vi "SentinelController v35 good v11.vi"() -> ()   [LabVIEW 2011] (continued)
                  n306 = local write "H1 Lock"(FALSE ("H1 Lock")) -> ()
                  n307 = local write "H2 warning 2"(FALSE ("H1 warning")) -> ()
                  n308 = local write "H2 warning"(FALSE ("H1 warning")) -> ()
                  n309 = local write "H1 warning 2"(FALSE ("H1 warning")) -> ()
                  n310 = local write "H1 warning"(FALSE ("H1 warning")) -> ()
                  n311 = local write "H2 nominal 2"(TRUE ("H1 nominal")) -> ()
                  n312 = local write "H2 alarm 2"(FALSE ("H1 warning")) -> ()
                  n313 = local write "H2 alarm"(FALSE ("H1 warning")) -> ()
                  n314 = local write "H1 nominal 2"(TRUE ("H1 nominal")) -> ()
                  n315 = local write "H1 alarm 2"(FALSE ("H1 warning")) -> ()
                  n316 = local write "system statuts hid"(T9."H1NH2N" ("system statuts")) -> ()
                  n317 = local write "H1 Good Units"(w3224) -> ()
                  n318 = local write "H2 Device Count"(w3224) -> ()
                  n319 = local write "H2 Good Units"(w3224) -> ()
                  n320 = local write "H1 Device Count"(w3224) -> ()
                  n321 = property on="System UPH" class="Knob (strict)"("Scale.Minimum"=w3221) -> ()  [unwired: 2 in, 2 out]
                  n322 = property on="H1 UPH" class="Knob (strict)"("Scale.Minimum"=w3221) -> ()  [unwired: 2 in, 2 out]
                  n323 = property on="H2 UPH" class="Knob (strict)"("Scale.Minimum"=w3221) -> ()  [unwired: 2 in, 2 out]
                  n324 = property on="SysUtilMon" class="WFChart (strict)"("History Data"=cluster{dbl, dbl}[] []) -> ()  [unwired: 2 in, 2 out]
                  n325 = local write "H1 alarm"(w3239) -> ()
                  n326 = local write "H2 alarm"(w3239) -> ()
                  n327 = property on="YieldMon" class="WFChart (strict)"("History Data"=cluster{dbl, dbl, dbl, dbl}[] []) -> ()  [unwired: 2 in, 2 out]
                  n328 = local write "YieldMon"(w3216) -> ()
                  n329 = local write "SysUtilMon"(w3215) -> ()
                  n330 = local write "Sys utilization"(0.0) -> ()
                  n331 = local write "H2 alarm 2"(w3239) -> ()
                  n332 = local write "H1 alarm 2"(w3239) -> ()
                  n333 = local write "H2 nominal"(TRUE ("H1 nominal")) -> ()
                  n334 = local write "H1 nominal"(TRUE ("H1 nominal")) -> ()
                  n335 = local read "Lot number"() -> (w3213:string)
                  n336 = local write "Number of text alerts"(0.0 ("Number of Emails Alerts Sent")) -> ()
                  n337 = local write "Number of email alerts"(u32 0 ("Number of Emails Alerts Sent")) -> ()
                  n338 = local write "Tester loop counter hid"(u32 0 ("Tester loop counter")) -> ()
                  n339 = local write "H1 loop counter hid"(u32 0 ("H1 loop counter hid")) -> ()
                  n340 = local write "H2 loop counter hid"(u32 0 ("H2 loop counter hid")) -> ()
                  n341 = local write "H1 Ready with sites"(FALSE ("H1 Ready with sites")) -> ()
                  n342 = local write "H2 Ready with sites"(FALSE ("H1 Ready with sites")) -> ()
                  n343 = local write "GPIB Bus 0 traffic"(w3218) -> ()
                  n344 = local write "Notifications Lot Display"(w3213) -> ()
                  n345 = local write "GPIB bus 1 traffic"(w3218) -> ()
                  n346 = local write "GPIB bus 2 traffic"(w3218) -> ()
                }
              }
              n347 = case shown="True" w3122 {
                frame False {
                }
                frame True {
                  w3198 = FALSE
                  n348 = local read "H1 online"() -> (w3200:bool)
                  n349 = local read "H2 online"() -> (w3199:bool)
                  n350 = Equal?(x=w3200, y=w3198) -> (x = y?=w3202:bool)
                  n351 = Equal?(x=w3198, y=w3199) -> (x = y?=w3201:bool)
                  n352 = Or(x=w3202, y=w3201) -> (x .or. y?=w3197:bool)
                  n353 = case shown="True" w3197 {
                    frame False {
                    }
                    frame True {
                      n354 = local write "Optimize handler speed"(FALSE ("Optimize Handler Speed")) -> ()
                    }
                  }
                }
              }
              n355 = local read "Alert volume"() -> (w3133:u32)
              n356 = Equal To 0?(x=w3133) -> (x = 0?=w3135:bool)
              n357 = case shown="True" w3135 {
                frame False {
                }
                frame True {
                  n358 = local write "Audio On / Off"(FALSE ("Audio On/Off")) -> ()
                }
              }
            }
            n359 = case shown="True" FALSE {
              frame False {
              }
              frame True {
                n360 = while {
                  i -> [w952]
                  stop <- w965 stop-if-true
                  # "Play Audio Aert Loop"
                  n361 = local read "Ignore alarms until AFTER this many cycles"() -> (w957:i32)
                  n362 = local read "H1 Device Count"() -> (w962:u32)
                  n363 = local read "H2 Device Count"() -> (w961:u32)
                  n364 = local read "Program Parallelism"() -> (w959:u32)
                  n365 = local read "Run"() -> (w954:bool)
                  n366 = local read "POWER"() -> (w955:bool)
                  n367 = Add(x=w962, y=w961) -> (x+y=w960:u32)
                  n368 = Wait (ms)(milliseconds to wait=u32 100) -> ()  [unwired: 1 out]
                  n369 = Divide(x=w960, y=w959) -> (x/y=w958:dbl)
                  n370 = Greater?(x=w952, y=50) -> (0:w950:bool)
                  n371 = Greater?(x=w958, y=w957) -> (0:w956:bool)
                  n372 = Compound Arithmetic op=AND(w956, w955, w954, w950) -> (w953:bool)
                  n373 = case shown="True" w953 {
                    frame False {
                    }
                    frame True {
                      n374 = local read "system statuts hid"() -> (w969:T9)
                      n375 = case shown="\"H1AH2A\"" w969 {
                        frame "H1NH2N", Default {
                          n376 = Wait (ms)(milliseconds to wait=u32 50) -> ()  [unwired: 1 out]
                        }
                        frame "H1NH2W" {
                          n377 = flat-sequence {
                            frame #0 {
                              n378 = local read "Audio On / Off"() -> (w972:bool)
                              n379 = local read "H2 online"() -> (w971:bool)
                              n380 = And(x=w971, y=w972) -> (x .and. y?=w973:bool)
                              n381 = case shown="True" w973 {
                                frame False {
                                }
                                frame True {
                                n382 = local read "Run"() -> (w976:bool)
                                n383 = case shown="True" w976 {
                                tunnel: [0.001 w978] -> w975
                                frame False {
                                }
                                frame True {
                                n384 = local read "Alert volume"() -> (w978:u32)
                                }
                                }
                                n385 = call "PlayAlarm.vi"("wavefilename"="audio\\4_synth_warning.wav", "alertvolume"=w975) -> ()  [unwired: 10 in]
                                }
                              }
                            }
                            frame #1 {
                              n386 = local read "Run"() -> (w979:bool)
                              n387 = case shown="True" w979 {
                                frame False {
                                }
                                frame True {
                                n388 = Wait (ms)(milliseconds to wait=u32 5000) -> ()  [unwired: 1 out]
                                }
                              }
                            }
                          }
                        }
                        frame "H1NH2A" {
                          n389 = flat-sequence {
                            frame #0 {
                              n390 = local read "Audio On / Off"() -> (w983:bool)
                              n391 = local read "H2 online"() -> (w982:bool)
                              n392 = And(x=w982, y=w983) -> (x .and. y?=w981:bool)
                              n393 = case shown="True" w981 {
                                frame False {
                                }
                                frame True {
                                n394 = local read "Run"() -> (w986:bool)
                                n395 = case shown="True" w986 {
                                tunnel: [0.001 w988] -> w985
                                frame False {
                                }
                                frame True {
                                n396 = local read "Alert volume"() -> (w988:u32)
                                }
                                }
                                n397 = call "PlayAlarm.vi"("wavefilename"="audio\\bass_synth_alarm.wav", "alertvolume"=w985) -> ()  [unwired: 10 in]
                                }
                              }
                            }
                            frame #1 {
                              n398 = local read "Run"() -> (w989:bool)
                              n399 = case shown="True" w989 {
                                frame False {
                                n400 = Wait (ms)(milliseconds to wait=u32 50) -> ()  [unwired: 1 out]
                                }
                                frame True {
                                n401 = Wait (ms)(milliseconds to wait=u32 5000) -> ()  [unwired: 1 out]
                                }
                              }
                            }
                          }
                        }
                        frame "H1WH2N" {
                          n402 = flat-sequence {
                            frame #0 {
                              n403 = local read "Audio On / Off"() -> (w994:bool)
                              n404 = local read "H1 online"() -> (w993:bool)
                              n405 = And(x=w993, y=w994) -> (x .and. y?=w992:bool)
                              n406 = case shown="True" w992 {
                                frame False {
                                }
                                frame True {
                                n407 = local read "Run"() -> (w997:bool)
                                n408 = case shown="True" w997 {
                                tunnel: [0.001 w999] -> w996
                                frame False {
                                }
                                frame True {
                                n409 = local read "Alert volume"() -> (w999:u32)
                                }
                                }
                                n410 = call "PlayAlarm.vi"("wavefilename"="audio\\4_synth_warning.wav", "alertvolume"=w996) -> ()  [unwired: 10 in]
                                }
                              }
                            }
                            frame #1 {
                              n411 = local read "Run"() -> (w1000:bool)
                              n412 = case shown="True" w1000 {
                                frame False {
                                n413 = Wait (ms)(milliseconds to wait=u32 50) -> ()  [unwired: 1 out]
                                }
                                frame True {
                                n414 = Wait (ms)(milliseconds to wait=u32 5000) -> ()  [unwired: 1 out]
                                }
                              }
                            }
                          }
                        }
                        frame "H1WH2W" {
                          n415 = flat-sequence {
                            frame #0 {
                              n416 = local read "Audio On / Off"() -> (w1006:bool)
                              n417 = local read "H1 online"() -> (w1003:bool)
                              n418 = local read "H2 online"() -> (w1005:bool)
                              n419 = Compound Arithmetic op=AND(w1003, w1005, w1006) -> (w1004:bool)
                              n420 = case shown="True" w1004 {
                                frame False {
                                }
                                frame True {
                                n421 = local read "Run"() -> (w1009:bool)
                                n422 = case shown="True" w1009 {
                                tunnel: [0.001 w1011] -> w1008
                                frame False {
                                }
                                frame True {
                                n423 = local read "Alert volume"() -> (w1011:u32)
                                }
                                }
                                n424 = call "PlayAlarm.vi"("wavefilename"="audio\\4_synth_warning.wav", "alertvolume"=w1008) -> ()  [unwired: 10 in]
                                }
                              }
                            }
                            frame #1 {
                              n425 = local read "Run"() -> (w1012:bool)
                              n426 = case shown="True" w1012 {
                                frame False {
                                n427 = Wait (ms)(milliseconds to wait=u32 50) -> ()  [unwired: 1 out]
                                }
                                frame True {
                                n428 = Wait (ms)(milliseconds to wait=u32 5000) -> ()  [unwired: 1 out]
                                }
                              }
                            }
                          }
                        }
                        frame "H1WH2A" {
                          n429 = flat-sequence {
                            frame #0 {
                              n430 = local read "Audio On / Off"() -> (w1018:bool)
                              n431 = local read "H1 online"() -> (w1016:bool)
                              n432 = local read "H2 online"() -> (w1017:bool)
                              n433 = Compound Arithmetic op=AND(w1016, w1017, w1018) -> (w1015:bool)
                              n434 = case shown="True" w1015 {
                                frame False {
                                }
                                frame True {
                                n435 = local read "Run"() -> (w1021:bool)
                                n436 = case shown="True" w1021 {
                                tunnel: [0.001 w1023] -> w1020
                                frame False {
                                }
                                frame True {
                                n437 = local read "Alert volume"() -> (w1023:u32)
                                }
                                }
                                n438 = call "PlayAlarm.vi"("wavefilename"="audio\\bass_synth_alarm.wav", "alertvolume"=w1020) -> ()  [unwired: 10 in]
                                }
                              }
                            }
                            frame #1 {
                              n439 = local read "Run"() -> (w1024:bool)
                              n440 = case shown="True" w1024 {
                                frame False {
                                n441 = Wait (ms)(milliseconds to wait=u32 50) -> ()  [unwired: 1 out]
                                }
                                frame True {
                                n442 = Wait (ms)(milliseconds to wait=u32 5000) -> ()  [unwired: 1 out]
                                }
                              }
                            }
                          }
                        }
                        frame "H1AH2N" {
                          n443 = flat-sequence {
                            frame #0 {
                              n444 = local read "Audio On / Off"() -> (w1029:bool)
                              n445 = local read "H1 online"() -> (w1027:bool)
                              n446 = And(x=w1027, y=w1029) -> (x .and. y?=w1028:bool)
                              n447 = case shown="True" w1028 {
                                frame False {
                                }
                                frame True {
                                n448 = local read "Run"() -> (w1032:bool)
                                n449 = case shown="True" w1032 {
                                tunnel: [0.001 w1034] -> w1031
                                frame False {
                                }
                                frame True {
                                n450 = local read "Alert volume"() -> (w1034:u32)
                                }
                                }
                                n451 = call "PlayAlarm.vi"("wavefilename"="audio\\bass_synth_alarm.wav", "alertvolume"=w1031) -> ()  [unwired: 10 in]
                                }
                              }
                            }
                            frame #1 {
                              n452 = local read "Run"() -> (w1035:bool)
                              n453 = case shown="True" w1035 {
                                frame False {
                                n454 = Wait (ms)(milliseconds to wait=u32 50) -> ()  [unwired: 1 out]
                                }
                                frame True {
                                n455 = Wait (ms)(milliseconds to wait=u32 5000) -> ()  [unwired: 1 out]
                                }
                              }
                            }
                          }
                        }
                        frame "H1AH2W" {
                          n456 = flat-sequence {
                            frame #0 {
                              n457 = local read "Audio On / Off"() -> (w1041:bool)
                              n458 = local read "H1 online"() -> (w1039:bool)
                              n459 = local read "H2 online"() -> (w1040:bool)
                              n460 = Compound Arithmetic op=AND(w1039, w1040, w1041) -> (w1038:bool)
                              n461 = case shown="True" w1038 {
                                frame False {
                                }
                                frame True {
                                n462 = local read "Run"() -> (w1044:bool)
                                n463 = case shown="True" w1044 {
                                tunnel: [0.001 w1046] -> w1043
                                frame False {
                                }
                                frame True {
                                n464 = local read "Alert volume"() -> (w1046:u32)
                                }
                                }
                                n465 = call "PlayAlarm.vi"("wavefilename"="audio\\bass_synth_alarm.wav", "alertvolume"=w1043) -> ()  [unwired: 10 in]
                                }
                              }
                            }
                            frame #1 {
                              n466 = local read "Run"() -> (w1047:bool)
                              n467 = case shown="True" w1047 {
                                frame False {
                                n468 = Wait (ms)(milliseconds to wait=u32 50) -> ()  [unwired: 1 out]
                                }
                                frame True {
                                n469 = Wait (ms)(milliseconds to wait=u32 5000) -> ()  [unwired: 1 out]
                                }
                              }
                            }
                          }
                        }
                        frame "H1AH2A" {
                          n470 = flat-sequence {
                            frame #0 {
                              n471 = local read "Audio On / Off"() -> (w1053:bool)
                              n472 = local read "H1 online"() -> (w1051:bool)
                              n473 = local read "H2 online"() -> (w1052:bool)
                              n474 = Compound Arithmetic op=AND(w1051, w1052, w1053) -> (w1050:bool)
                              n475 = case shown="True" w1050 {
                                frame False {
                                }
                                frame True {
                                n476 = local read "Run"() -> (w1056:bool)
                                n477 = case shown="True" w1056 {
                                tunnel: [0.001 w1058] -> w1055
                                frame False {
                                }
                                frame True {
                                n478 = local read "Alert volume"() -> (w1058:u32)
                                }
                                }
                                n479 = call "PlayAlarm.vi"("wavefilename"="audio\\bass_synth_alarm.wav", "alertvolume"=w1055) -> ()  [unwired: 10 in]
                                }
                              }
                            }
                            frame #1 {
                              n480 = local read "Run"() -> (w1059:bool)
                              n481 = case shown="True" w1059 {
                                frame False {
                                n482 = Wait (ms)(milliseconds to wait=u32 50) -> ()  [unwired: 1 out]
                                }
                                frame True {
                                n483 = Wait (ms)(milliseconds to wait=u32 5000) -> ()  [unwired: 1 out]
                                }
                              }
                            }
                          }
                        }
                      }
                    }
                  }
                  n484 = local read "Run"() -> (w963:bool)
                  n485 = local read "POWER"() -> (w966:bool)
                  n486 = Not(x=w966) -> (.not. x?=w968:bool)
                  n487 = Not(x=w963) -> (.not. x?=w967:bool)
                  n488 = Compound Arithmetic op=OR(w968, w967) -> (w965:bool)
                }
              }
            }
            n489 = while {
              shift-right: [w2528] -> _
              shift-left: T9."H1NH2N" ("system statuts") -> [w2518]
              stop <- w2517 continue-if-true
              # "system status state machine:\n- writes data log whenever there is a change (if data loggin enabled)\n- issues email and text alerts is enabled (electronic notification of alarms)"
              n490 = local read "H1 parallelism"() -> (w2524:u32)
              n491 = local read "H1 Device Count"() -> (w2525:u32)
              n492 = local read "H2 Device Count"() -> (w2523:u32)
              n493 = local read "H2 parallelism"() -> (w2522:u32)
              n494 = local read "POWER"() -> (w2517:bool)
              n495 = Divide(x=w2523, y=w2522) -> (x/y=w2519:dbl)
              n496 = Divide(x=w2525, y=w2524) -> (x/y=w2520:dbl)
              n497 = local read "Ignore alarms until AFTER this many cycles"() -> (w2527:i32)
              n498 = Add(x=w2520, y=w2519) -> (x+y=w2521:dbl)
              n499 = Greater?(x=w2521, y=w2527) -> (0:w2526:bool)
              n500 = case shown="True" w2526 {
                tunnel: [w2530 w2533] -> w2528
                tunnel: w2518 -> [w2530 w2531]
                frame False {
                }
                frame True {
                  n501 = flat-sequence {
                    tunnel: [w2534] -> w2532
                    tunnel: w2531 -> [w2534]
                    tunnel: [w2631] -> w2533
                    tunnel: w2532 -> [w2629]
                    frame #0 {
                      # "Determine current state for System Status state-machine"
                      n502 = stacked-sequence {
                        frame #0 {
                          n503 = local read "H1 nominal 2"() -> (w2538:bool)
                          n504 = local read "H2 nominal 2"() -> (w2536:bool)
                          n505 = local read "H1 nominal"() -> (w2539:bool)
                          n506 = local read "H2 nominal"() -> (w2537:bool)
                          n507 = Compound Arithmetic op=AND(w2539, w2538, w2537, w2536) -> (w2535:bool)
                          n508 = case shown="True" w2535 {
                            frame False {
                            }
                            frame True {
                              n509 = local write "system statuts hid"(T9."H1NH2N" ("system statuts")) -> ()
                            }
                          }
                        }
                        frame #1 {
                          n510 = local read "H2 warning 2"() -> (w2543:bool)
                          n511 = local read "H2 warning"() -> (w2544:bool)
                          n512 = local read "H1 nominal 2"() -> (w2545:bool)
                          n513 = local read "H1 nominal"() -> (w2546:bool)
                          n514 = Or(x=w2544, y=w2543) -> (x .or. y?=w2542:bool)
                          n515 = Compound Arithmetic op=AND(w2546, w2545, w2542) -> (w2541:bool)
                          n516 = case shown="False" w2541 {
                            frame False {
                            }
                            frame True {
                              n517 = local write "system statuts hid"(T9."H1NH2W" ("system statuts")) -> ()
                            }
                          }
                        }
                        frame #2 {
                          n518 = local read "H1 nominal 2"() -> (w2553:bool)
                          n519 = local read "H1 nominal"() -> (w2554:bool)
                          n520 = local read "H2 alarm 2"() -> (w2551:bool)
                          n521 = local read "H2 alarm"() -> (w2552:bool)
                          n522 = Or(x=w2552, y=w2551) -> (x .or. y?=w2549:bool)
                          n523 = And(x=w2554, y=w2553) -> (x .and. y?=w2550:bool)
                          n524 = And(x=w2550, y=w2549) -> (x .and. y?=w2548:bool)
                          n525 = case shown="True" w2548 {
                            frame False {
                            }
                            frame True {
                              n526 = local write "system statuts hid"(T9."H1NH2A" ("system statuts")) -> ()
                            }
                          }
                        }
                        frame #3 {
                          n527 = local read "H1 alarm 2"() -> (w2564:bool)
                          n528 = local read "H1 alarm"() -> (w2565:bool)
                          n529 = local read "H2 nominal 2"() -> (w2567:bool)
                          n530 = local read "H1 warning 2"() -> (w2560:bool)
                          n531 = local read "H1 warning"() -> (w2561:bool)
                          n532 = local read "H2 nominal"() -> (w2566:bool)
                          n533 = Not(x=w2565) -> (.not. x?=w2563:bool)
                          n534 = Not(x=w2564) -> (.not. x?=w2562:bool)
                          n535 = Or(x=w2561, y=w2560) -> (x .or. y?=w2558:bool)
                          n536 = And(x=w2563, y=w2562) -> (x .and. y?=w2557:bool)
                          n537 = And(x=w2566, y=w2567) -> (x .and. y?=w2556:bool)
                          n538 = Compound Arithmetic op=AND(w2558, w2557, w2556) -> (w2559:bool)
                          n539 = case shown="True" w2559 {
                            frame False {
                            }
                            frame True {
                              n540 = local write "system statuts hid"(T9."H1WH2N" ("system statuts")) -> ()
                            }
                          }
                        }
                        frame #4 {
                          n541 = local read "H1 alarm 2"() -> (w2579:bool)
                          n542 = local read "H2 alarm 2"() -> (w2584:bool)
                          n543 = local read "H1 alarm"() -> (w2578:bool)
                          n544 = local read "H2 alarm"() -> (w2585:bool)
                          n545 = local read "H1 warning 2"() -> (w2575:bool)
                          n546 = local read "H2 warning 2"() -> (w2576:bool)
                          n547 = local read "H1 warning"() -> (w2574:bool)
                          n548 = local read "H2 warning"() -> (w2577:bool)
                          n549 = Not(x=w2578) -> (.not. x?=w2580:bool)
                          n550 = Not(x=w2579) -> (.not. x?=w2581:bool)
                          n551 = Not(x=w2585) -> (.not. x?=w2583:bool)
                          n552 = Not(x=w2584) -> (.not. x?=w2582:bool)
                          n553 = Or(x=w2574, y=w2575) -> (x .or. y?=w2572:bool)
                          n554 = Or(x=w2577, y=w2576) -> (x .or. y?=w2570:bool)
                          n555 = And(x=w2580, y=w2581) -> (x .and. y?=w2571:bool)
                          n556 = And(x=w2583, y=w2582) -> (x .and. y?=w2569:bool)
                          n557 = Compound Arithmetic op=AND(w2572, w2571, w2570, w2569) -> (w2573:bool)
                          n558 = case shown="True" w2573 {
                            frame False {
                            }
                            frame True {
                              n559 = local write "system statuts hid"(T9."H1WH2W" ("system statuts")) -> ()
                            }
                          }
                        }
                        frame #5 {
                          n560 = local read "H1 alarm 2"() -> (w2592:bool)
                          n561 = local read "H1 alarm"() -> (w2593:bool)
                          n562 = local read "H1 warning 2"() -> (w2595:bool)
                          n563 = local read "H1 warning"() -> (w2596:bool)
                          n564 = local read "H2 alarm 2"() -> (w2597:bool)
                          n565 = local read "H2 alarm"() -> (w2598:bool)
                          n566 = Not(x=w2593) -> (.not. x?=w2591:bool)
                          n567 = Not(x=w2592) -> (.not. x?=w2590:bool)
                          n568 = Or(x=w2596, y=w2595) -> (x .or. y?=w2589:bool)
                          n569 = Or(x=w2598, y=w2597) -> (x .or. y?=w2587:bool)
                          n570 = And(x=w2591, y=w2590) -> (x .and. y?=w2588:bool)
                          n571 = Compound Arithmetic op=AND(w2589, w2588, w2587) -> (w2594:bool)
                          n572 = case shown="True" w2594 {
                            frame False {
                            }
                            frame True {
                              n573 = local write "system statuts hid"(T9."H1WH2A" ("system statuts")) -> ()
                            }
                          }
                        }
                        frame #6 {
                          n574 = local read "H2 nominal 2"() -> (w2605:bool)
                          n575 = local read "H2 nominal"() -> (w2606:bool)
                          n576 = local read "H1 alarm 2"() -> (w2603:bool)
                          n577 = local read "H1 alarm"() -> (w2604:bool)
                          n578 = Or(x=w2604, y=w2603) -> (x .or. y?=w2601:bool)
                          n579 = And(x=w2606, y=w2605) -> (x .and. y?=w2600:bool)
                          n580 = And(x=w2601, y=w2600) -> (x .and. y?=w2602:bool)
                          n581 = case shown="True" w2602 {
                            frame False {
                            }
                            frame True {
                              n582 = local write "system statuts hid"(T9."H1AH2N" ("system statuts")) -> ()
                            }
                          }
                        }
                        frame #7 {
                          n583 = local read "H2 alarm 2"() -> (w2610:bool)
                          n584 = local read "H2 alarm"() -> (w2611:bool)
                          n585 = local read "H2 warning 2"() -> (w2616:bool)
                          n586 = local read "H2 warning"() -> (w2617:bool)
                          n587 = local read "H1 alarm 2"() -> (w2618:bool)
                          n588 = local read "H1 alarm"() -> (w2619:bool)
                          n589 = Not(x=w2611) -> (.not. x?=w2609:bool)
                          n590 = Not(x=w2610) -> (.not. x?=w2608:bool)
                          n591 = Or(x=w2619, y=w2618) -> (x .or. y?=w2614:bool)
                          n592 = Or(x=w2617, y=w2616) -> (x .or. y?=w2613:bool)
                          n593 = And(x=w2609, y=w2608) -> (x .and. y?=w2612:bool)
                          n594 = Compound Arithmetic op=AND(w2614, w2613, w2612) -> (w2615:bool)
                          n595 = case shown="True" w2615 {
                            frame False {
                            }
                            frame True {
                              n596 = local write "system statuts hid"(T9."H1AH2W" ("system statuts")) -> ()
                            }
                          }
                        }
                        frame #8 {
                          n597 = local read "H1 alarm 2"() -> (w2625:bool)
                          n598 = local read "H2 alarm 2"() -> (w2624:bool)
                          n599 = local read "H1 alarm"() -> (w2626:bool)
                          n600 = local read "H2 alarm"() -> (w2623:bool)
                          n601 = Or(x=w2626, y=w2625) -> (x .or. y?=w2621:bool)
                          n602 = Or(x=w2623, y=w2624) -> (x .or. y?=w2622:bool)
                          n603 = And(x=w2621, y=w2622) -> (x .and. y?=w2627:bool)
                          n604 = case shown="True" w2627 {
                            frame False {
                            }
                            frame True {
                              n605 = local write "system statuts hid"(T9."H1AH2A" ("system statuts")) -> ()
                            }
                          }
                        }
                      }
                    }
                    frame #1 {
                      n606 = local read "system statuts hid"() -> (w2631:T9)
                      n607 = Not Equal?(x=w2631, y=w2629) -> (x != y?=w2630:bool)
                      n608 = case shown="True" w2630 {
                        tunnel: w2631 -> [_ w2633]
                        frame False {
                        }
                        frame True {
                          n609 = local read "Enable data logging of all events"() -> (w2632:bool)
                          n610 = case shown="True" w2632 {
                            tunnel: w2633 -> [_ w2634]
                            frame False {
                            }
                            frame True {
                              n611 = stacked-sequence {
                                tunnel: w2634 -> [_ w2637 _ _ _]
                                frame #0 {
                                n612 = local read "Number of data log entries hid"() -> (w2636:u32)
                                n613 = Increment(x=w2636) -> (x+1=w2635:u32)
                                n614 = local write "Number of data log entries hid"(w2635) -> ()
                                }
                                frame #1 {
                                n615 = case shown="\"H1AH2A\"" w2637 {
                                frame "H1NH2N", Default {
                                w2644 = "\r\n"
                                n616 = local read "H1 online"() -> (w2661:bool)
                                n617 = local read "H2 online"() -> (w2662:bool)
                                n618 = local read "Number of data log entries hid"() -> (w2638:u32)
                                n619 = local read "H1 UPH warning limit hid"() -> (w2657:dbl)
                                n620 = local read "H2 UPH warning limit hid"() -> (w2659:dbl)
                                n621 = local read "YieldMon"() -> (w2642:cluster{i32, i32, i32, i32})
                                n622 = local read "H2  low yield warning"() -> (w2658:dbl)
                                n623 = local read "H1 low yield warning"() -> (w2656:dbl)
                                n624 = local read "H1 UPH"() -> (w2650:cluster{u32, u32})
                                n625 = local read "H2 UPH"() -> (w2648:cluster{u32, u32})
                                n626 = local read "YieldMon"() -> (w2640:cluster{i32, i32, i32, i32})
                                n627 = case shown="True" w2661 {
                                tunnel: ["H1 Off-Line" "H1 On-Line"] -> w2663
                                frame False {
                                }
                                frame True {
                                }
                                }
                                n628 = case shown="True" w2662 {
                                tunnel: ["H2 Off-Line" "H2 On-Line"] -> w2672
                                frame False {
                                }
                                frame True {
                                }
                                }
                                n629 = Unbundle(w2642) -> (w2641:i32)  [unwired: 3 out]
                                n630 = Unbundle(w2650) -> (w2649:u32)  [unwired: 1 out]
                                n631 = Unbundle(w2640) -> (w2639:i32)  [unwired: 3 out]
                                n632 = Unbundle(w2648) -> (w2647:u32)  [unwired: 1 out]
                                n633 = local read "Data log path and filename"() -> (w2646:path)
                                n634 = Number To Decimal String(number=w2656) -> (decimal integer string=w2665:string)  [unwired: 1 in]
                                n635 = Number To Decimal String(number=w2641) -> (decimal integer string=w2667:string)  [unwired: 1 in]
                                n636 = Number To Decimal String(number=w2657) -> (decimal integer string=w2669:string)  [unwired: 1 in]
                                n637 = Number To Decimal String(number=w2649) -> (decimal integer string=w2671:string)  [unwired: 1 in]
                                n638 = Number To Decimal String(number=w2658) -> (decimal integer string=w2674:string)  [unwired: 1 in]
                                n639 = Number To Decimal String(number=w2639) -> (decimal integer string=w2676:string)  [unwired: 1 in]
                                n640 = Number To Decimal String(number=w2659) -> (decimal integer string=w2678:string)  [unwired: 1 in]
                                n641 = Number To Decimal String(number=w2647) -> (decimal integer string=w2680:string)  [unwired: 1 in]
                                n642 = Number To Decimal String(number=w2638) -> (decimal integer string=w2643:string)  [unwired: 1 in]
                                n643 = Get Date/Time String(want seconds? (F)=TRUE) -> (date string=w2654:string, time string=w2655:string)  [unwired: 2 in]
                                n644 = Concatenate Strings(w2643, w2644, w2654, "   " ("string"), w2655, w2644, "H1 Nominal, H2 Nominal", w2644, w2663, w2644, "H1 Low Yield Warning Limit: ", w2665, ", H1 yield = ", w2667, w2644, "H1 Low UPH Warning Limit: ", w2669, ", H1 UPH = ", w2671, w2644, w2672, w2644, "H2 Low Yield Warning Limit: ", w2674, ", H2 yield = ", w2676, w2644, "H2 Low UPH Warning Limit: ", w2678, ", H2 UPH = ", w2680, w2644, w2644) -> (w2652:string)
                                n645 = call "SentinelDatalog.vi"("operation (0:open)"=T10."open", "String"=w2652, "data log path"=w2646) -> ()  [unwired: 8 in, 1 out]
                                }
                                frame "H1NH2W" {
                                w2690 = "\r\n"
                                n646 = local read "H1 online"() -> (w2708:bool)
                                n647 = local read "H2 online"() -> (w2709:bool)
                                n648 = local read "H1 UPH warning limit hid"() -> (w2704:dbl)
                                n649 = local read "H2 UPH warning limit hid"() -> (w2706:dbl)
                                n650 = local read "YieldMon"() -> (w2689:cluster{i32, i32, i32, i32})
                                n651 = local read "H2  low yield warning"() -> (w2705:dbl)
                                n652 = local read "H1 low yield warning"() -> (w2703:dbl)
                                n653 = local read "H1 UPH"() -> (w2697:cluster{u32, u32})
                                n654 = local read "H2 UPH"() -> (w2695:cluster{u32, u32})
                                n655 = local read "YieldMon"() -> (w2687:cluster{i32, i32, i32, i32})
                                n656 = local read "Number of data log entries hid"() -> (w2685:u32)
                                n657 = case shown="True" w2708 {
                                tunnel: ["H1 Off-Line" "H1 On-Line"] -> w2710
                                frame False {
                                }
                                frame True {
                                }
                                }
                                n658 = case shown="True" w2709 {
                                tunnel: ["H2 Off-Line" "H2 On-Line"] -> w2719
                                frame False {
                                }
                                frame True {
                                }
                                }
                                n659 = Unbundle(w2687) -> (w2686:i32)  [unwired: 3 out]
                                n660 = Unbundle(w2697) -> (w2696:u32)  [unwired: 1 out]
                                n661 = Unbundle(w2689) -> (w2688:i32)  [unwired: 3 out]
                                n662 = Unbundle(w2695) -> (w2694:u32)  [unwired: 1 out]
                                n663 = Number To Decimal String(number=w2703) -> (decimal integer string=w2712:string)  [unwired: 1 in]
                                n664 = Number To Decimal String(number=w2686) -> (decimal integer string=w2714:string)  [unwired: 1 in]
                                n665 = Number To Decimal String(number=w2704) -> (decimal integer string=w2716:string)  [unwired: 1 in]
                                n666 = Number To Decimal String(number=w2696) -> (decimal integer string=w2718:string)  [unwired: 1 in]
                                n667 = Number To Decimal String(number=w2705) -> (decimal integer string=w2721:string)  [unwired: 1 in]
                                n668 = Number To Decimal String(number=w2688) -> (decimal integer string=w2723:string)  [unwired: 1 in]
                                n669 = Number To Decimal String(number=w2706) -> (decimal integer string=w2725:string)  [unwired: 1 in]
                                n670 = Number To Decimal String(number=w2694) -> (decimal integer string=w2727:string)  [unwired: 1 in]
                                n671 = Number To Decimal String(number=w2685) -> (decimal integer string=w2691:string)  [unwired: 1 in]
                                n672 = local read "Data log path and filename"() -> (w2693:path)
                                n673 = Get Date/Time String(want seconds? (F)=TRUE) -> (date string=w2701:string, time string=w2702:string)  [unwired: 2 in]
                                n674 = Concatenate Strings(w2691, w2690, w2701, "   " ("string"), w2702, w2690, "H1 Nominal, H2 Warning", w2690, w2710, w2690, "H1 Low Yield Warning Limit: ", w2712, ", H1 yield = ", w2714, w2690, "H1 Low UPH Warning Limit: ", w2716, ", H1 UPH = ", w2718, w2690, w2719, w2690, "H2 Low Yield Warning Limit: ", w2721, ", H2 yield = ", w2723, w2690, "H2 Low UPH Warning Limit: ", w2725, ", H2 UPH = ", w2727, w2690, w2690) -> (w2699:string)
                                n675 = call "SentinelDatalog.vi"("operation (0:open)"=T10."open", "String"=w2699, "data log path"=w2693) -> ()  [unwired: 8 in, 1 out]
                                }
                                frame "H1NH2A" {
                                w2738 = "\r\n"
                                n676 = local read "H1 online"() -> (w2755:bool)
                                n677 = local read "H2 online"() -> (w2756:bool)
                                n678 = local read "Number of data log entries hid"() -> (w2732:u32)
                                n679 = local read "H1 UPH warning limit hid"() -> (w2751:dbl)
                                n680 = local read "H1 low yield warning"() -> (w2750:dbl)
                                n681 = local read "H2 UPH alarm limit hid"() -> (w2753:dbl)
                                n682 = local read "YieldMon"() -> (w2736:cluster{i32, i32, i32, i32})
                                n683 = local read "H1 UPH"() -> (w2744:cluster{u32, u32})
                                n684 = local read "H2 low yield alarm"() -> (w2752:dbl)
                                n685 = local read "H2 UPH"() -> (w2743:cluster{u32, u32})
                                n686 = local read "YieldMon"() -> (w2734:cluster{i32, i32, i32, i32})
                                n687 = case shown="True" w2755 {
                                tunnel: ["H1 Off-Line" "H1 On-Line"] -> w2757
                                frame False {
                                }
                                frame True {
                                }
                                }
                                n688 = case shown="True" w2756 {
                                tunnel: ["H2 Off-Line" "H2 On-Line"] -> w2766
                                frame False {
                                }
                                frame True {
                                }
                                }
                                n689 = Number To Decimal String(number=w2732) -> (decimal integer string=w2737:string)  [unwired: 1 in]
                                n690 = Unbundle(w2736) -> (w2735:i32)  [unwired: 3 out]
                                n691 = Unbundle(w2744) -> (w2741:u32)  [unwired: 1 out]
                                n692 = Unbundle(w2734) -> (w2733:i32)  [unwired: 3 out]
                                n693 = Unbundle(w2743) -> (w2742:u32)  [unwired: 1 out]
                                n694 = Number To Decimal String(number=w2750) -> (decimal integer string=w2759:string)  [unwired: 1 in]
                                n695 = Number To Decimal String(number=w2735) -> (decimal integer string=w2761:string)  [unwired: 1 in]
                                n696 = Number To Decimal String(number=w2751) -> (decimal integer string=w2763:string)  [unwired: 1 in]
                                n697 = Number To Decimal String(number=w2741) -> (decimal integer string=w2765:string)  [unwired: 1 in]
                                n698 = Number To Decimal String(number=w2752) -> (decimal integer string=w2768:string)  [unwired: 1 in]
                                n699 = Number To Decimal String(number=w2733) -> (decimal integer string=w2770:string)  [unwired: 1 in]
                                n700 = Number To Decimal String(number=w2753) -> (decimal integer string=w2772:string)  [unwired: 1 in]
                                n701 = Number To Decimal String(number=w2742) -> (decimal integer string=w2774:string)  [unwired: 1 in]
                                n702 = local read "Data log path and filename"() -> (w2740:path)
                                n703 = Get Date/Time String(want seconds? (F)=TRUE) -> (date string=w2748:string, time string=w2749:string)  [unwired: 2 in]
                                n704 = Concatenate Strings(w2737, w2738, w2748, "   " ("string"), w2749, w2738, "H1 Nominal, H2 Alarming", w2738, w2757, w2738, "H1 Low Yield Warning Limit: ", w2759, ", H1 yield = ", w2761, w2738, "H1 Low UPH Warning Limit: ", w2763, ", H1 UPH = ", w2765, w2738, w2766, w2738, "H2 Low Yield Alarm Limit: ", w2768, ", H2 yield = ", w2770, w2738, "H2 Low UPH Alarm Limit: ", w2772, ", H2 UPH = ", w2774, w2738, w2738) -> (w2746:string)
                                n705 = call "SentinelDatalog.vi"("operation (0:open)"=T10."open", "String"=w2746, "data log path"=w2740) -> ()  [unwired: 8 in, 1 out]
                                }
                                frame "H1WH2N" {
                                w2785 = "\r\n"
                                n706 = local read "H1 online"() -> (w2803:bool)
                                n707 = local read "H2 online"() -> (w2804:bool)
                                n708 = local read "H1 UPH warning limit hid"() -> (w2799:dbl)
                                n709 = local read "H2 UPH warning limit hid"() -> (w2801:dbl)
                                n710 = local read "H2  low yield warning"() -> (w2800:dbl)
                                n711 = local read "H1 low yield warning"() -> (w2798:dbl)
                                n712 = local read "H1 UPH"() -> (w2791:cluster{u32, u32})
                                n713 = local read "H2 UPH"() -> (w2790:cluster{u32, u32})
                                n714 = local read "YieldMon"() -> (w2783:cluster{i32, i32, i32, i32})
                                n715 = local read "YieldMon"() -> (w2781:cluster{i32, i32, i32, i32})
                                n716 = local read "Number of data log entries hid"() -> (w2779:u32)
                                n717 = case shown="True" w2803 {
                                tunnel: ["H1 Off-Line" "H1 On-Line"] -> w2792
                                frame False {
                                }
                                frame True {
                                }
                                }
                                n718 = case shown="True" w2804 {
                                tunnel: ["H2 Off-Line" "H2 On-Line"] -> w2813
                                frame False {
                                }
                                frame True {
                                }
                                }
                                n719 = Unbundle(w2783) -> (w2782:i32)  [unwired: 3 out]
                                n720 = Unbundle(w2791) -> (w2788:u32)  [unwired: 1 out]
                                n721 = Unbundle(w2781) -> (w2780:i32)  [unwired: 3 out]
                                n722 = Unbundle(w2790) -> (w2789:u32)  [unwired: 1 out]
                                n723 = Number To Decimal String(number=w2798) -> (decimal integer string=w2806:string)  [unwired: 1 in]
                                n724 = Number To Decimal String(number=w2782) -> (decimal integer string=w2808:string)  [unwired: 1 in]
                                n725 = Number To Decimal String(number=w2799) -> (decimal integer string=w2810:string)  [unwired: 1 in]
                                n726 = Number To Decimal String(number=w2788) -> (decimal integer string=w2812:string)  [unwired: 1 in]
                                n727 = Number To Decimal String(number=w2800) -> (decimal integer string=w2815:string)  [unwired: 1 in]
                                n728 = Number To Decimal String(number=w2780) -> (decimal integer string=w2817:string)  [unwired: 1 in]
                                n729 = Number To Decimal String(number=w2801) -> (decimal integer string=w2819:string)  [unwired: 1 in]
                                n730 = Number To Decimal String(number=w2789) -> (decimal integer string=w2821:string)  [unwired: 1 in]
                                n731 = local read "Data log path and filename"() -> (w2787:path)
                                n732 = Number To Decimal String(number=w2779) -> (decimal integer string=w2784:string)  [unwired: 1 in]
                                n733 = Get Date/Time String(want seconds? (F)=TRUE) -> (date string=w2796:string, time string=w2797:string)  [unwired: 2 in]
                                n734 = Concatenate Strings(w2784, w2785, w2796, "   " ("string"), w2797, w2785, "H1 Warning, H2 Nominal", w2785, w2792, w2785, "H1 Low Yield Warning Limit: ", w2806, ", H1 yield = ", w2808, w2785, "H1 Low UPH Warning Limit: ", w2810, ", H1 UPH = ", w2812, w2785, w2813, w2785, "H2 Low Yield Warning Limit: ", w2815, ", H2 yield = ", w2817, w2785, "H2 Low UPH Warning Limit: ", w2819, ", H2 UPH = ", w2821, w2785, w2785) -> (w2794:string)
                                n735 = call "SentinelDatalog.vi"("operation (0:open)"=T10."open", "String"=w2794, "data log path"=w2787) -> ()  [unwired: 8 in, 1 out]
                                }
                                frame "H1WH2W" {
                                w2831 = "\r\n"
                                w2839 = "\r\n"
                                n736 = local read "H1 online"() -> (w2850:bool)
                                n737 = local read "H2 online"() -> (w2851:bool)
                                n738 = local read "H1 UPH warning limit hid"() -> (w2846:dbl)
                                n739 = local read "H2 UPH warning limit hid"() -> (w2848:dbl)
                                n740 = local read "H2  low yield warning"() -> (w2847:dbl)
                                n741 = local read "H1 low yield warning"() -> (w2845:dbl)
                                n742 = local read "H1 UPH"() -> (w2838:cluster{u32, u32})
                                n743 = local read "H2 UPH"() -> (w2837:cluster{u32, u32})
                                n744 = local read "YieldMon"() -> (w2830:cluster{i32, i32, i32, i32})
                                n745 = local read "YieldMon"() -> (w2828:cluster{i32, i32, i32, i32})
                                n746 = case shown="True" w2850 {
                                tunnel: ["H1 Off-Line" "H1 On-Line"] -> w2852
                                frame False {
                                }
                                frame True {
                                }
                                }
                                n747 = case shown="True" w2851 {
                                tunnel: ["H2 Off-Line" "H2 On-Line"] -> w2861
                                frame False {
                                }
                                frame True {
                                }
                                }
                                n748 = local read "Number of data log entries hid"() -> (w2826:u32)
                                n749 = Unbundle(w2830) -> (w2829:i32)  [unwired: 3 out]
                                n750 = Unbundle(w2838) -> (w2836:u32)  [unwired: 1 out]
                                n751 = Unbundle(w2828) -> (w2827:i32)  [unwired: 3 out]
                                n752 = Unbundle(w2837) -> (w2835:u32)  [unwired: 1 out]
                                n753 = Number To Decimal String(number=w2845) -> (decimal integer string=w2854:string)  [unwired: 1 in]
                                n754 = Number To Decimal String(number=w2829) -> (decimal integer string=w2856:string)  [unwired: 1 in]
                                n755 = Number To Decimal String(number=w2846) -> (decimal integer string=w2858:string)  [unwired: 1 in]
                                n756 = Number To Decimal String(number=w2836) -> (decimal integer string=w2860:string)  [unwired: 1 in]
                                n757 = Number To Decimal String(number=w2847) -> (decimal integer string=w2863:string)  [unwired: 1 in]
                                n758 = Number To Decimal String(number=w2827) -> (decimal integer string=w2865:string)  [unwired: 1 in]
                                n759 = Number To Decimal String(number=w2848) -> (decimal integer string=w2867:string)  [unwired: 1 in]
                                n760 = Number To Decimal String(number=w2835) -> (decimal integer string=w2869:string)  [unwired: 1 in]
                                n761 = local read "Data log path and filename"() -> (w2834:path)
                                n762 = Get Date/Time String(want seconds? (F)=TRUE) -> (date string=w2843:string, time string=w2844:string)  [unwired: 2 in]
                                n763 = Number To Decimal String(number=w2826) -> (decimal integer string=w2832:string)  [unwired: 1 in]
                                n764 = Concatenate Strings(w2832, w2831, w2843, "   " ("string"), w2844, w2831, "H1 Warning, H2 Warning", w2831, w2852, w2831, "H1 Low Yield Warning Limit: ", w2854, ", H1 yield = ", w2856, w2839, "H1 Low UPH Warning Limit: ", w2858, ", H1 UPH = ", w2860, w2839, w2861, w2839, "H2 Low Yield Warning Limit: ", w2863, ", H2 yield = ", w2865, w2839, "H2 Low UPH Warning Limit: ", w2867, ", H2 UPH = ", w2869, w2839, w2839) -> (w2841:string)
                                n765 = call "SentinelDatalog.vi"("operation (0:open)"=T10."open", "String"=w2841, "data log path"=w2834) -> ()  [unwired: 8 in, 1 out]
                                }
                                frame "H1WH2A" {
                                w2880 = "\r\n"
                                n766 = local read "H1 online"() -> (w2897:bool)
                                n767 = local read "H2 online"() -> (w2898:bool)
                                n768 = local read "H1 UPH warning limit hid"() -> (w2893:dbl)
                                n769 = local read "H1 low yield warning"() -> (w2892:dbl)
                                n770 = local read "H2 UPH alarm limit hid"() -> (w2895:dbl)
                                n771 = local read "H1 UPH"() -> (w2886:cluster{u32, u32})
                                n772 = local read "H2 low yield alarm"() -> (w2894:dbl)
                                n773 = local read "H2 UPH"() -> (w2885:cluster{u32, u32})
                                n774 = local read "YieldMon"() -> (w2876:cluster{i32, i32, i32, i32})
                                n775 = local read "YieldMon"() -> (w2878:cluster{i32, i32, i32, i32})
                                n776 = local read "Number of data log entries hid"() -> (w2874:u32)
                                n777 = case shown="True" w2897 {
                                tunnel: ["H1 Off-Line" "H1 On-Line"] -> w2899
                                frame False {
                                }
                                frame True {
                                }
                                }
                                n778 = case shown="True" w2898 {
                                tunnel: ["H2 Off-Line" "H2 On-Line"] -> w2908
                                frame False {
                                }
                                frame True {
                                }
                                }
                                n779 = Unbundle(w2876) -> (w2875:i32)  [unwired: 3 out]
                                n780 = Unbundle(w2886) -> (w2884:u32)  [unwired: 1 out]
                                n781 = Unbundle(w2878) -> (w2877:i32)  [unwired: 3 out]
                                n782 = Unbundle(w2885) -> (w2883:u32)  [unwired: 1 out]
                                n783 = Number To Decimal String(number=w2892) -> (decimal integer string=w2901:string)  [unwired: 1 in]
                                n784 = Number To Decimal String(number=w2875) -> (decimal integer string=w2903:string)  [unwired: 1 in]
                                n785 = Number To Decimal String(number=w2893) -> (decimal integer string=w2905:string)  [unwired: 1 in]
                                n786 = Number To Decimal String(number=w2884) -> (decimal integer string=w2907:string)  [unwired: 1 in]
                                n787 = Number To Decimal String(number=w2894) -> (decimal integer string=w2910:string)  [unwired: 1 in]
                                n788 = Number To Decimal String(number=w2877) -> (decimal integer string=w2912:string)  [unwired: 1 in]
                                n789 = Number To Decimal String(number=w2895) -> (decimal integer string=w2914:string)  [unwired: 1 in]
                                n790 = Number To Decimal String(number=w2883) -> (decimal integer string=w2916:string)  [unwired: 1 in]
                                n791 = local read "Data log path and filename"() -> (w2882:path)
                                n792 = Get Date/Time String(want seconds? (F)=TRUE) -> (date string=w2890:string, time string=w2891:string)  [unwired: 2 in]
                                n793 = Number To Decimal String(number=w2874) -> (decimal integer string=w2879:string)  [unwired: 1 in]
